vi "NKTP_API_VITree.vi"   [LabVIEW 2011, in "NKTP_API.lvlib"]
uses:
  <instrlib>/NKTP_API/NKTP_API.lvlib
panel:
  # "All VIs in the NKTP LabVIEW API  is located on the block diagram -->>\nYou can drag and drop API VIs from there to your own diagrams"
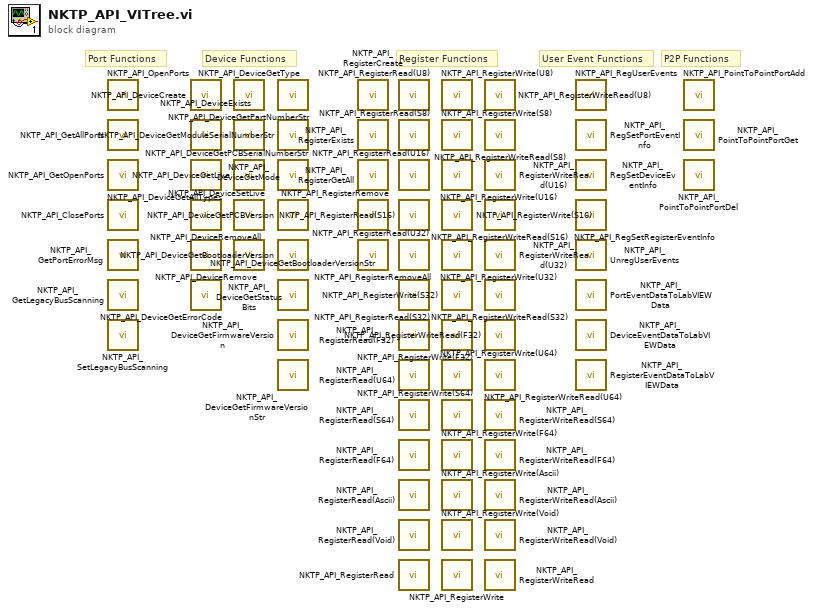
[diagram p0: block diagram]
diagram:
  # "P2P Functions"
  # "Register Functions"
  # "Port Functions"
  # "User Event Functions"
  # "Device Functions"
  n1 = call <instrlib>:"NKTP_API_OpenPorts.vi"() -> ()  [unwired: 10 in, 2 out]
  n2 = call <instrlib>:"NKTP_API_GetAllPorts.vi"() -> ()  [unwired: 10 in, 2 out]
  n3 = call <instrlib>:"NKTP_API_GetOpenPorts.vi"() -> ()  [unwired: 10 in, 2 out]
  n4 = call <instrlib>:"NKTP_API_ClosePorts.vi"() -> ()  [unwired: 10 in, 2 out]
  n5 = call <instrlib>:"NKTP_API_GetPortErrorMsg.vi"() -> ()  [unwired: 9 in, 3 out]
  n6 = call <instrlib>:"NKTP_API_GetLegacyBusScanning.vi"() -> ()  [unwired: 9 in, 3 out]
  n7 = call <instrlib>:"NKTP_API_SetLegacyBusScanning.vi"() -> ()  [unwired: 10 in, 2 out]
  n8 = call <instrlib>:"NKTP_API_DeviceCreate.vi"() -> ()  [unwired: 10 in, 2 out]
  n9 = call <instrlib>:"NKTP_API_DeviceExists.vi"() -> ()  [unwired: 9 in, 3 out]
  n10 = call <instrlib>:"NKTP_API_DeviceGetAllTypes.vi"() -> ()  [unwired: 9 in, 3 out]
  n11 = call <instrlib>:"NKTP_API_DeviceRemoveAll.vi"() -> ()  [unwired: 10 in, 2 out]
  n12 = call <instrlib>:"NKTP_API_DeviceRemove.vi"() -> ()  [unwired: 10 in, 2 out]
  n13 = call <instrlib>:"NKTP_API_DeviceGetErrorCode.vi"() -> ()  [unwired: 9 in, 3 out]
  n14 = call <instrlib>:"NKTP_API_DeviceGetType.vi"() -> ()  [unwired: 9 in, 3 out]
  n15 = call <instrlib>:"NKTP_API_DeviceGetMode.vi"() -> ()  [unwired: 9 in, 3 out]
  n16 = call <instrlib>:"NKTP_API_DeviceGetLive.vi"() -> ()  [unwired: 9 in, 3 out]
  n17 = call <instrlib>:"NKTP_API_DeviceSetLive.vi"() -> ()  [unwired: 10 in, 2 out]
  n18 = call <instrlib>:"NKTP_API_DeviceGetStatusBits.vi"() -> ()  [unwired: 9 in, 3 out]
  n19 = call <instrlib>:"NKTP_API_DeviceGetPartNumberStr.vi"() -> ()  [unwired: 9 in, 3 out]
  n20 = call <instrlib>:"NKTP_API_DeviceGetModuleSerialNumberStr.vi"() -> ()  [unwired: 9 in, 3 out]
  n21 = call <instrlib>:"NKTP_API_DeviceGetPCBSerialNumberStr.vi"() -> ()  [unwired: 9 in, 3 out]
  n22 = call <instrlib>:"NKTP_API_DeviceGetPCBVersion.vi"() -> ()  [unwired: 9 in, 3 out]
  n23 = call <instrlib>:"NKTP_API_DeviceGetBootloaderVersion.vi"() -> ()  [unwired: 9 in, 3 out]
  n24 = call <instrlib>:"NKTP_API_DeviceGetBootloaderVersionStr.vi"() -> ()  [unwired: 9 in, 3 out]
  n25 = call <instrlib>:"NKTP_API_DeviceGetFirmwareVersion.vi"() -> ()  [unwired: 9 in, 3 out]
  n26 = call <instrlib>:"NKTP_API_DeviceGetFirmwareVersionStr.vi"() -> ()  [unwired: 9 in, 3 out]
  n27 = call <instrlib>:"NKTP_API_RegisterCreate.vi"() -> ()  [unwired: 10 in, 2 out]
  n28 = call <instrlib>:"NKTP_API_RegisterExists.vi"() -> ()  [unwired: 9 in, 3 out]
  n29 = call <instrlib>:"NKTP_API_RegisterGetAll.vi"() -> ()  [unwired: 9 in, 3 out]
  n30 = call <instrlib>:"NKTP_API_RegisterRemove.vi"() -> ()  [unwired: 10 in, 2 out]
  n31 = call <instrlib>:"NKTP_API_RegisterRemoveAll.vi"() -> ()  [unwired: 10 in, 2 out]
  n32 = call <instrlib>:"NKTP_API_RegisterRead(U8).vi"() -> ()  [unwired: 9 in, 3 out]
  n33 = call <instrlib>:"NKTP_API_RegisterRead(S8).vi"() -> ()  [unwired: 9 in, 3 out]
  n34 = call <instrlib>:"NKTP_API_RegisterRead(U16).vi"() -> ()  [unwired: 9 in, 3 out]
  n35 = call <instrlib>:"NKTP_API_RegisterRead(S16).vi"() -> ()  [unwired: 9 in, 3 out]
  n36 = call <instrlib>:"NKTP_API_RegisterRead(U32).vi"() -> ()  [unwired: 9 in, 3 out]
  n37 = call <instrlib>:"NKTP_API_RegisterRead(S32).vi"() -> ()  [unwired: 9 in, 3 out]
  n38 = call <instrlib>:"NKTP_API_RegisterRead(F32).vi"() -> ()  [unwired: 9 in, 3 out]
  n39 = call <instrlib>:"NKTP_API_RegisterRead(U64).vi"() -> ()  [unwired: 9 in, 3 out]
  n40 = call <instrlib>:"NKTP_API_RegisterRead(S64).vi"() -> ()  [unwired: 9 in, 3 out]
  n41 = call <instrlib>:"NKTP_API_RegisterRead(F64).vi"() -> ()  [unwired: 9 in, 3 out]
  n42 = call <instrlib>:"NKTP_API_RegisterRead(Ascii).vi"() -> ()  [unwired: 8 in, 4 out]
  n43 = call <instrlib>:"NKTP_API_RegisterRead(Void).vi"() -> ()  [unwired: 8 in, 4 out]
  n44 = call-poly <instrlib>:"NKTP_API_RegisterRead.vi"() -> ()  [unwired: 8 in, 4 out]
  n45 = call <instrlib>:"NKTP_API_RegisterWrite(U8).vi"() -> ()  [unwired: 10 in, 2 out]
  n46 = call <instrlib>:"NKTP_API_RegisterWrite(S8).vi"() -> ()  [unwired: 10 in, 2 out]
  n47 = call <instrlib>:"NKTP_API_RegisterWrite(U16).vi"() -> ()  [unwired: 10 in, 2 out]
  n48 = call <instrlib>:"NKTP_API_RegisterWrite(S16).vi"() -> ()  [unwired: 10 in, 2 out]
  n49 = call <instrlib>:"NKTP_API_RegisterWrite(U32).vi"() -> ()  [unwired: 10 in, 2 out]
  n50 = call <instrlib>:"NKTP_API_RegisterWrite(S32).vi"() -> ()  [unwired: 10 in, 2 out]
  n51 = call <instrlib>:"NKTP_API_RegisterWrite(F32).vi"() -> ()  [unwired: 10 in, 2 out]
  n52 = call <instrlib>:"NKTP_API_RegisterWrite(U64).vi"() -> ()  [unwired: 10 in, 2 out]
  n53 = call <instrlib>:"NKTP_API_RegisterWrite(S64).vi"() -> ()  [unwired: 10 in, 2 out]
  n54 = call <instrlib>:"NKTP_API_RegisterWrite(F64).vi"() -> ()  [unwired: 10 in, 2 out]
  n55 = call <instrlib>:"NKTP_API_RegisterWrite(Ascii).vi"() -> ()  [unwired: 10 in, 2 out]
  n56 = call <instrlib>:"NKTP_API_RegisterWrite(Void).vi"() -> ()  [unwired: 10 in, 2 out]
  n57 = call-poly <instrlib>:"NKTP_API_RegisterWrite.vi"() -> ()  [unwired: 10 in, 2 out]
  n58 = call <instrlib>:"NKTP_API_RegisterWriteRead(U8).vi"() -> ()  [unwired: 9 in, 3 out]
  n59 = call <instrlib>:"NKTP_API_RegisterWriteRead(S8).vi"() -> ()  [unwired: 9 in, 3 out]
  n60 = call <instrlib>:"NKTP_API_RegisterWriteRead(U16).vi"() -> ()  [unwired: 9 in, 3 out]
  n61 = call <instrlib>:"NKTP_API_RegisterWriteRead(S16).vi"() -> ()  [unwired: 9 in, 3 out]
  n62 = call <instrlib>:"NKTP_API_RegisterWriteRead(U32).vi"() -> ()  [unwired: 9 in, 3 out]
  n63 = call <instrlib>:"NKTP_API_RegisterWriteRead(S32).vi"() -> ()  [unwired: 9 in, 3 out]
  n64 = call <instrlib>:"NKTP_API_RegisterWriteRead(F32).vi"() -> ()  [unwired: 9 in, 3 out]
  n65 = call <instrlib>:"NKTP_API_RegisterWriteRead(U64).vi"() -> ()  [unwired: 9 in, 3 out]
  n66 = call <instrlib>:"NKTP_API_RegisterWriteRead(S64).vi"() -> ()  [unwired: 9 in, 3 out]
  n67 = call <instrlib>:"NKTP_API_RegisterWriteRead(F64).vi"() -> ()  [unwired: 9 in, 3 out]
  n68 = call <instrlib>:"NKTP_API_RegisterWriteRead(Ascii).vi"() -> ()  [unwired: 8 in, 4 out]
  n69 = call <instrlib>:"NKTP_API_RegisterWriteRead(Void).vi"() -> ()  [unwired: 8 in, 4 out]
  n70 = call-poly <instrlib>:"NKTP_API_RegisterWriteRead.vi"() -> ()  [unwired: 8 in, 4 out]
  n71 = call <instrlib>:"NKTP_API_RegUserEvents.vi"() -> ()  [unwired: 7 in, 5 out]
  n72 = call <instrlib>:"NKTP_API_RegSetPortEventInfo.vi"() -> ()  [unwired: 10 in, 2 out]
  n73 = call <instrlib>:"NKTP_API_RegSetDeviceEventInfo.vi"() -> ()  [unwired: 10 in, 2 out]
  n74 = call <instrlib>:"NKTP_API_RegSetRegisterEventInfo.vi"() -> ()  [unwired: 10 in, 2 out]
  n75 = call <instrlib>:"NKTP_API_UnregUserEvents.vi"() -> ()  [unwired: 11 in, 1 out]
  n76 = call <instrlib>:"NKTP_API_PortEventDataToLabVIEWData.vi"() -> ()  [unwired: 10 in, 2 out]
  n77 = call <instrlib>:"NKTP_API_DeviceEventDataToLabVIEWData.vi"() -> ()  [unwired: 10 in, 2 out]
  n78 = call <instrlib>:"NKTP_API_RegisterEventDataToLabVIEWData.vi"() -> ()  [unwired: 9 in, 3 out]
  n79 = call <instrlib>:"NKTP_API_PointToPointPortAdd.vi"() -> ()  [unwired: 10 in, 2 out]
  n80 = call <instrlib>:"NKTP_API_PointToPointPortGet.vi"() -> ()  [unwired: 6 in, 6 out]
  n81 = call <instrlib>:"NKTP_API_PointToPointPortDel.vi"() -> ()  [unwired: 9 in, 3 out]
